vi "FGV Hover Preview.vi"(9 "Mouse Coordinates":T1, 10 "Net Data":T4, 11 "Command":enum16{"Open", "Close", "Tick"}(ring)) -> ()   [LabVIEW 2019]
uses:
  Advanced Search.llb/Terminal Filter Output.ctl
  Advanced Search.llb/Terminals within Selection and GObject.ctl
  <vilib>/Utility/miscctls.llb/LVPoint32TypeDef.ctl
  Hover Preview Data.ctl
panel:
  out "VI Information":string
  out "2D Picture":picture
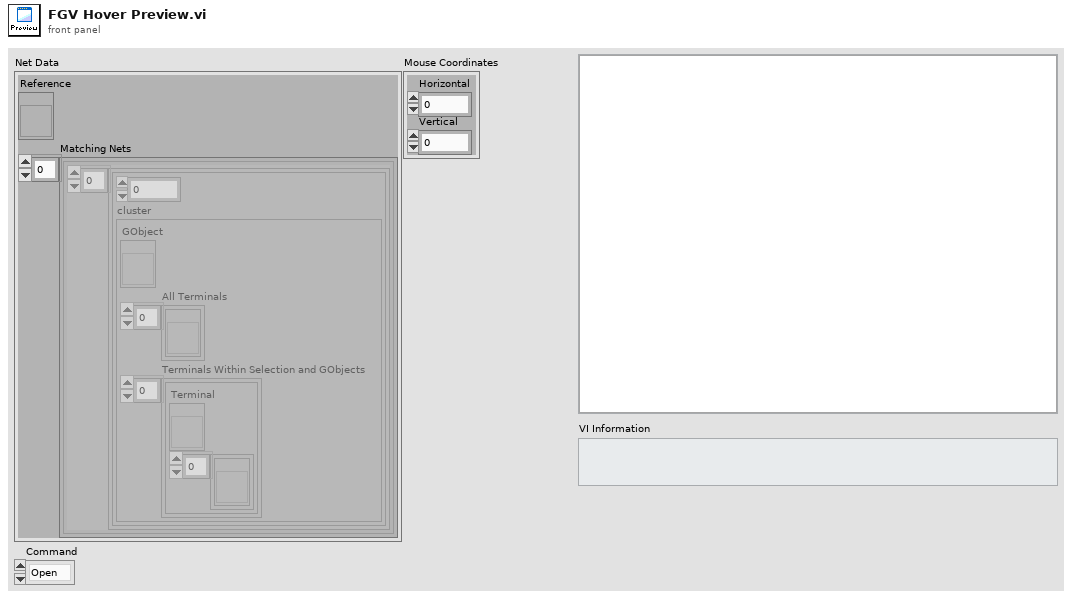
[diagram p1: front panel]
types:
  T1 = typedef "LVPoint32TypeDef.ctl" = cluster{"Horizontal":i32, "Vertical":i32}
  T2 = typedef "Terminal Filter Output.ctl" = cluster{"GObject":refnum<vi>, "All Terminals":refnum<vi>[], "Terminals Within Selection and GObjects":T3[]}
  T3 = typedef "Terminals within Selection and GObject.ctl" = cluster{"Terminal":refnum<vi>, "Attached GObjects":refnum<vi>[]}
  T4 = cluster{"Reference":refnum<vi>, "Matching Nets":cluster{cluster{i32, "cluster":T2}[]}[]}
  T5 = typedef "Hover Preview Data.ctl" = cluster{"Net Data":cluster{"Reference":refnum<vi>, "Matching Nets":cluster{cluster{i32, "cluster":T2}[]}[]}, "Current Net Index":i32, "Last Preview Change":u32}
  T6 = typedef "imagedata.ctl" = cluster{"image type":i32, "image depth":i32, "image":u8[], "mask":u8[], "colors":u32[], "Rectangle":cluster{"left":i16, "top":i16, "right":i16, "bottom":i16}}
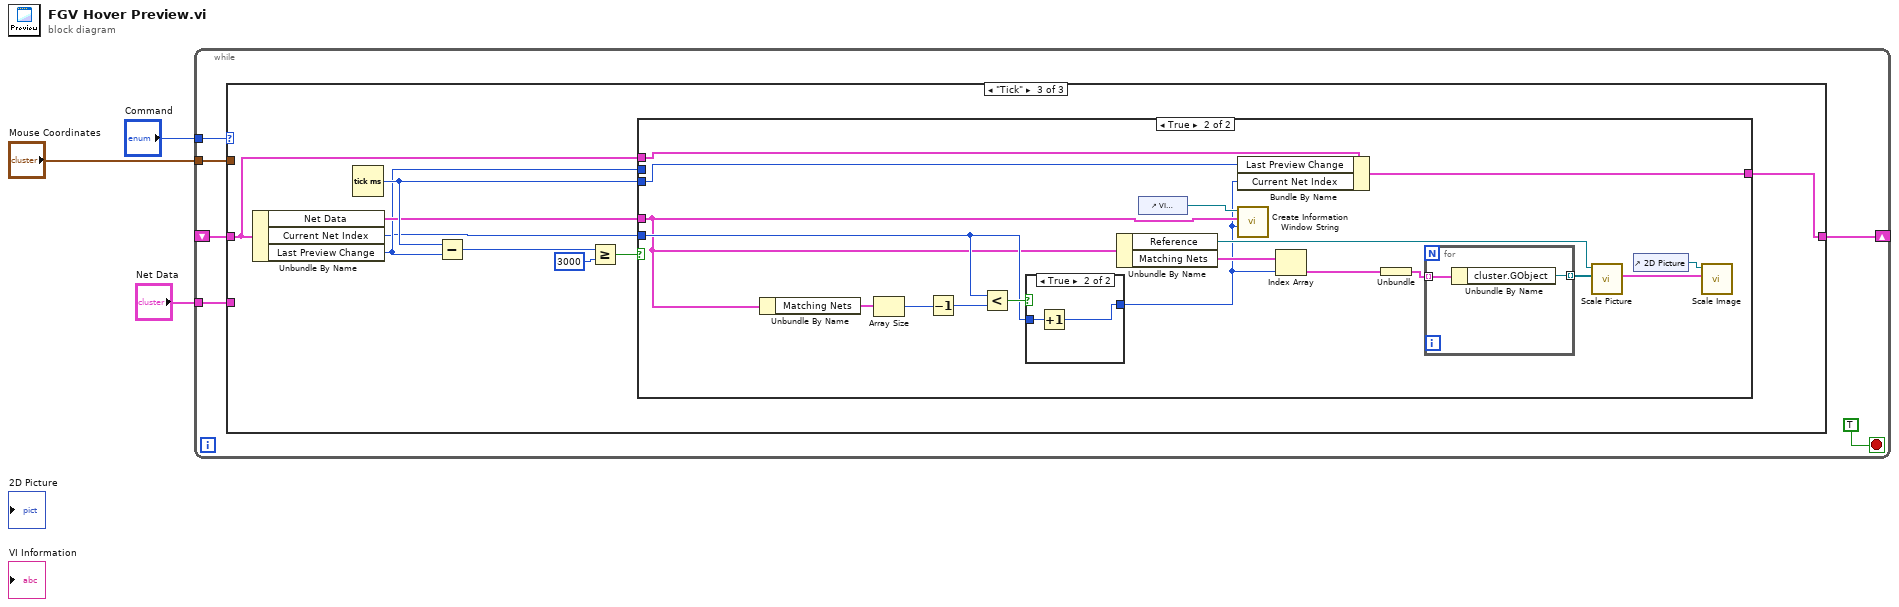
[diagram p0: block diagram]
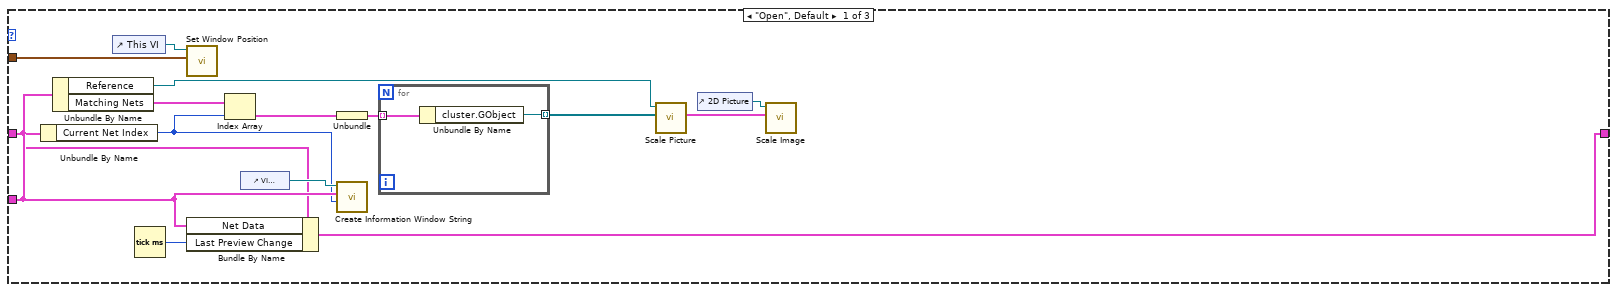
[diagram p2: hidden frame]
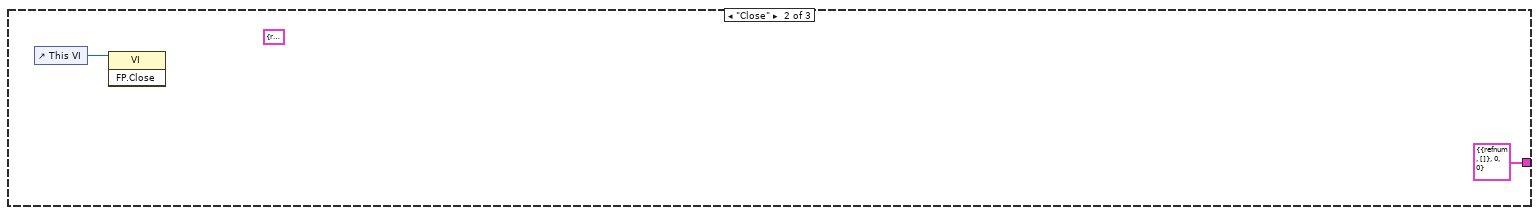
[diagram p3: hidden frame]
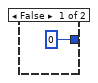
[diagram p5: hidden frame]
diagram:
  n1 = while {
    tunnel: "Command" -> [w8]
    tunnel: "Net Data" -> [w7]
    tunnel: "Mouse Coordinates" -> [w6]
    shift-right: [w5] -> _
    shift-left: _ -> [w4]
    stop <- TRUE stop-if-true
    n2 = case shown="\"Tick\"" w8 {
      tunnel: w7 -> [w12 _ _]
      tunnel: w6 -> [w18 _ _]
      tunnel: [w14 T5 {"Net Data"={"Reference"=refnum, "Matching Nets"=[]}, "Current Net Index"=0, "Last Preview Change"=0} w30] -> w5
      tunnel: w4 -> [w11 _ w29]
      frame "Open", Default {
        n3 = Unbundle By Name(w11) -> ("Current Net Index"=w10:i32)
        n4 = Unbundle By Name(w12) -> ("Reference"=w15:refnum<vi>, "Matching Nets"=w16:cluster{cluster{i32, "cluster":T2}[]}[])
        n5 = control-ref of="This VI"() -> (w19:refnum<vi>)
        n6 = Tick Count (ms)() -> (millisecond timer value=w13:u32)
        n7 = call "Set Window Position.vi"("Mouse Coordinates"=w18, "VI in"=w19) -> ()  [unwired: 9 in, 1 out]
        n8 = Bundle By Name(cluster=w11, "Net Data"=w12, "Last Preview Change"=w13) -> (w14:T5)
        n9 = Index Array(array=w16, index=w10) -> (element=w24:cluster{cluster{i32, "cluster":T2}[]})
        n10 = control-ref of="VI Information"() -> (w17:refnum<vi>)
        n11 = Unbundle(w24) -> (w23:cluster{i32, "cluster":T2}[])
        n12 = call "Create Information Window String.vi"("Current Network Index"=w10, "Net Data"=w12, "Information Window Reference"=w17) -> ()  [unwired: 9 in]
        n13 = for {
          tunnel: w23 -> [w26] mode=indexing
          tunnel: [w25] -> w22 mode=indexing
          n14 = Unbundle By Name(w26) -> ("cluster.GObject"=w25:refnum<vi>)
        }
        n15 = call "Scale Picture.vi"("Refnums 1"=w22, "VI in"=w15) -> ("image subset"=w21:T6)  [unwired: 8 in, 1 out]
        n16 = control-ref of="2D Picture"() -> (w20:refnum<vi>)
        n17 = call "Scale Image.vi"("Selected Data"=w21, "Picture in"=w20) -> ()  [unwired: 9 in, 1 out]
      }
      frame "Close" {
        (unwired) T4 {"Reference"=refnum, "Matching Nets"=[]} ("Net Data")
        n18 = control-ref of="This VI"() -> (w28:refnum<vi>)
        n19 = invoke class="VI" method="FP.Close"(reference=w28) -> ()  [unwired: 2 in, 3 out]
      }
      frame "Tick" {
        n20 = Unbundle By Name(w29) -> ("Net Data"=w33:T4, "Current Net Index"=w31:i32, "Last Preview Change"=w32:u32)
        n21 = Tick Count (ms)() -> (millisecond timer value=w34:u32)
        n22 = Subtract(x=w34, y=w32) -> (x-y=w37:u32)
        n23 = Greater Or Equal?(x=w37, y=u32 3000) -> (x >= y?=w35:bool)
        n24 = case shown="True" w35 {
          tunnel: w33 -> [_ w45]
          tunnel: w31 -> [_ w47]
          tunnel: w34 -> [_ w40]
          tunnel: w32 -> [_ _]
          tunnel: [w38 w41] -> w30
          tunnel: w29 -> [w38 w42]
          frame False {
          }
          frame True {
            n25 = Unbundle By Name(w45) -> ("Matching Nets"=w43:cluster{cluster{i32, "cluster":T2}[]}[])
            n26 = Array Size(array=w43) -> (size(s)=w56:i32)
            n27 = Decrement(x=w56) -> (x-1=w46:i32)
            n28 = Less?(x=w47, y=w46) -> (x < y?=w55:bool)
            n29 = case shown="True" w55 {
              tunnel: [0 w60] -> w39
              tunnel: w47 -> [_ w61]
              frame False {
              }
              frame True {
                n30 = Increment(x=w61) -> (x+1=w60:i32)
              }
            }
            n31 = Unbundle By Name(w45) -> ("Reference"=w48:refnum<vi>, "Matching Nets"=w49:cluster{cluster{i32, "cluster":T2}[]}[])
            n32 = control-ref of="VI Information"() -> (w44:refnum<vi>)
            n33 = Bundle By Name(cluster=w42, "Last Preview Change"=w40, "Current Net Index"=w39) -> (w41:T5)
            n34 = call "Create Information Window String.vi"("Current Network Index"=w39, "Net Data"=w45, "Information Window Reference"=w44) -> ()  [unwired: 9 in]
            n35 = Index Array(array=w49, index=w39) -> (element=w50:cluster{cluster{i32, "cluster":T2}[]})
            n36 = Unbundle(w50) -> (w51:cluster{i32, "cluster":T2}[])
            n37 = for {
              tunnel: w51 -> [w58] mode=indexing
              tunnel: [w57] -> w52 mode=indexing
              n38 = Unbundle By Name(w58) -> ("cluster.GObject"=w57:refnum<vi>)
            }
            n39 = call "Scale Picture.vi"("Refnums 1"=w52, "VI in"=w48) -> ("image subset"=w53:T6)  [unwired: 8 in, 1 out]
            n40 = control-ref of="2D Picture"() -> (w54:refnum<vi>)
            n41 = call "Scale Image.vi"("Selected Data"=w53, "Picture in"=w54) -> ()  [unwired: 9 in, 1 out]
          }
        }
      }
    }
  }
